vi "process output.vi"(8 "error in":errorcluster, 9 "result allocation":T1, 10 "parameters":T1, 11 "module in":refnum<class "current tag file io module runtime.lvclass">) -> (0 "error out":errorcluster, 1 "results":T1, 2 "parameter allocation":T1, 3 "module out":refnum<class "current tag file io module runtime.lvclass">)   [LabVIEW 2013, in "current tag file io module runtime.lvclass"]
doc: "Provides an interface for information processing by a module at runtime. While this interface performs no operations, a child should provide an override which may process data in any manner necessary."
uses:
  current tag file io module runtime.lvclass
  <vilib>/NI/Tag Bus/table/data table.lvlib
  <vilib>/NI/Tag Bus/table/data polymorphs/read one/read Double.vi
  <vilib>/NI/Tag Bus/table/data polymorphs/write one/write Double.vi
  <vilib>/NI/Tag Bus/table/data polymorphs/read one/read Boolean.vi
  <vilib>/NI/Tag Bus/table/data polymorphs/write one/write Array of String.vi
  <vilib>/NI/Tag Bus/table/data polymorphs/read one/read Array of String.vi
  <vilib>/NI/Tag Bus/table/data polymorphs/read one/read Single.vi
  <vilib>/NI/Tag Bus/table/data polymorphs/write one/write Single.vi
  <vilib>/NI/Tag Bus/table/data polymorphs/read one/read I64.vi
  <vilib>/NI/Tag Bus/table/data polymorphs/write one/write I64.vi
  <vilib>/NI/Tag Bus/table/data polymorphs/read one/read I32.vi
  <vilib>/NI/Tag Bus/table/data polymorphs/write one/write I32.vi
  <vilib>/NI/Tag Bus/table/data polymorphs/read one/read I16.vi
  <vilib>/NI/Tag Bus/table/data polymorphs/write one/write I16.vi
  <vilib>/NI/Tag Bus/table/data polymorphs/read one/read I8.vi
  <vilib>/NI/Tag Bus/table/data polymorphs/write one/write I8.vi
  <vilib>/NI/Tag Bus/table/data polymorphs/read one/read U64.vi
  <vilib>/NI/Tag Bus/table/data polymorphs/write one/write U64.vi
  <vilib>/NI/Tag Bus/table/data polymorphs/read one/read U32.vi
  <vilib>/NI/Tag Bus/table/data polymorphs/write one/write U32.vi
  <vilib>/NI/Tag Bus/table/data polymorphs/read one/read U16.vi
  <vilib>/NI/Tag Bus/table/data polymorphs/write one/write U16.vi
  <vilib>/NI/Tag Bus/table/data polymorphs/read one/read U8.vi
  <vilib>/NI/Tag Bus/table/data polymorphs/write one/write U8.vi
  <vilib>/NI/Tag Bus/table/data polymorphs/write one/write Boolean.vi
  <vilib>/NI/Tag Bus/table/data polymorphs/read one/read String.vi
  <vilib>/NI/Tag Bus/table/data polymorphs/write one/write String.vi
  <vilib>/NI/Tag Bus/table/data polymorphs/read one/read Array of Double.vi
  <vilib>/NI/Tag Bus/table/data polymorphs/write one/write Array of Double.vi
  <vilib>/NI/Tag Bus/table/data polymorphs/read one/read Array of Single.vi
  <vilib>/NI/Tag Bus/table/data polymorphs/write one/write Array of Single.vi
  <vilib>/NI/Tag Bus/table/data polymorphs/read one/read Array of I64.vi
  <vilib>/NI/Tag Bus/table/data polymorphs/write one/write Array of I64.vi
  <vilib>/NI/Tag Bus/table/data polymorphs/read one/read Array of I32.vi
  <vilib>/NI/Tag Bus/table/data polymorphs/write one/write Array of I32.vi
  <vilib>/NI/Tag Bus/table/data polymorphs/read one/read Array of I16.vi
  <vilib>/NI/Tag Bus/table/data polymorphs/write one/write Array of I16.vi
  <vilib>/NI/Tag Bus/table/data polymorphs/read one/read Array of I8.vi
  <vilib>/NI/Tag Bus/table/data polymorphs/write one/write Array of I8.vi
  <vilib>/NI/Tag Bus/table/data polymorphs/read one/read Array of U64.vi
  <vilib>/NI/Tag Bus/table/data polymorphs/write one/write Array of U64.vi
  <vilib>/NI/Tag Bus/table/data polymorphs/read one/read Array of U32.vi
  <vilib>/NI/Tag Bus/table/data polymorphs/write one/write Array of U32.vi
  <vilib>/NI/Tag Bus/table/data polymorphs/read one/read Array of U16.vi
  <vilib>/NI/Tag Bus/table/data polymorphs/write one/write Array of U16.vi
  <vilib>/NI/Tag Bus/table/data polymorphs/read one/read Array of U8.vi
  <vilib>/NI/Tag Bus/table/data polymorphs/write one/write Array of U8.vi
  <vilib>/NI/Tag Bus/table/data polymorphs/read one/read Array of Boolean.vi
  <vilib>/NI/Tag Bus/table/data polymorphs/write one/write Array of Boolean.vi
  <vilib>/NI/Tag Bus/table/data table.ctl
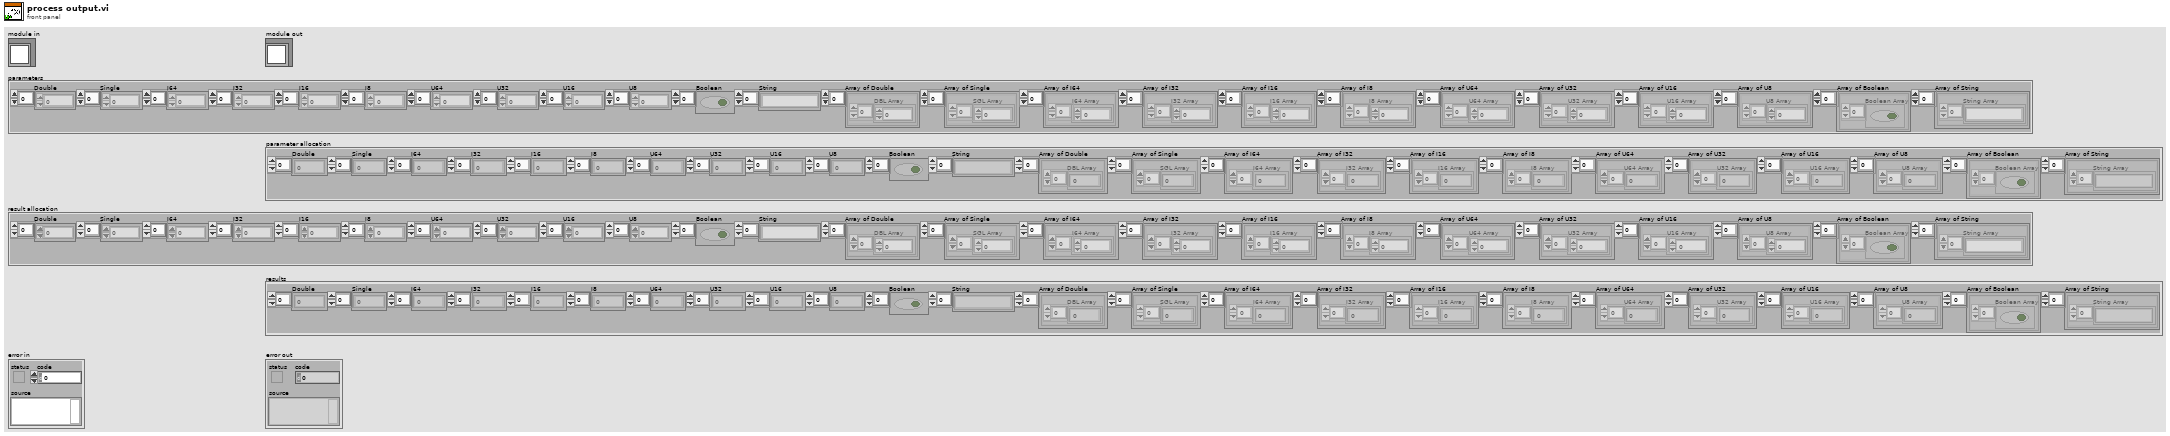
[diagram p1: front panel]
types:
  T1 = typedef "tag bus.lvlib/data table.lvlib/data table.ctl" = cluster{"Double":dbl[], "Single":sgl[], "I64":i64[], "I32":i32[], "I16":i16[], "I8":i8[], "U64":u64[], "U32":u32[], "U16":u16[], "U8":u8[], "Boolean":bool[], "String":string[], "Array of Double":cluster{"DBL Array":dbl[]}[], "Array of Single":cluster{"SGL Array":sgl[]}[], "Array of I64":cluster{"I64 Array":i64[]}[], "Array of I32":cluster{"I32 Array":i32[]}[], "Array of I16":cluster{"I16 Array":i16[]}[], "Array of I8":cluster{"I8 Array":i8[]}[], "Array of U64":cluster{"U64 Array":u64[]}[], "Array of U32":cluster{"U32 Array":u32[]}[], "Array of U16":cluster{"U16 Array":u16[]}[], "Array of U8":cluster{"U8 Array":u8[]}[], "Array of Boolean":cluster{"Boolean Array":bool[]}[], "Array of String":cluster{"String Array":string[]}[]}
  T2 = typedef "current tag file io module runtime.lvclass/runtime tag select configuration.ctl" = cluster{"channel index":i32, "data type":T3}
  T3 = typedef "tag bus.lvlib/tag descriptor.lvclass/Data Type.ctl" = enum16{"Double", "Single", "I64", "I32", "I16", "I8", "U64", "U32", "U16", "U8", "Boolean", "String", "Array of Double", "Array of Single", "Array of I64", "Array of I32", "Array of I16", "Array of I8", "Array of U64", "Array of U32", "Array of U16", "Array of U8", "Array of Boolean", "Array of String"}
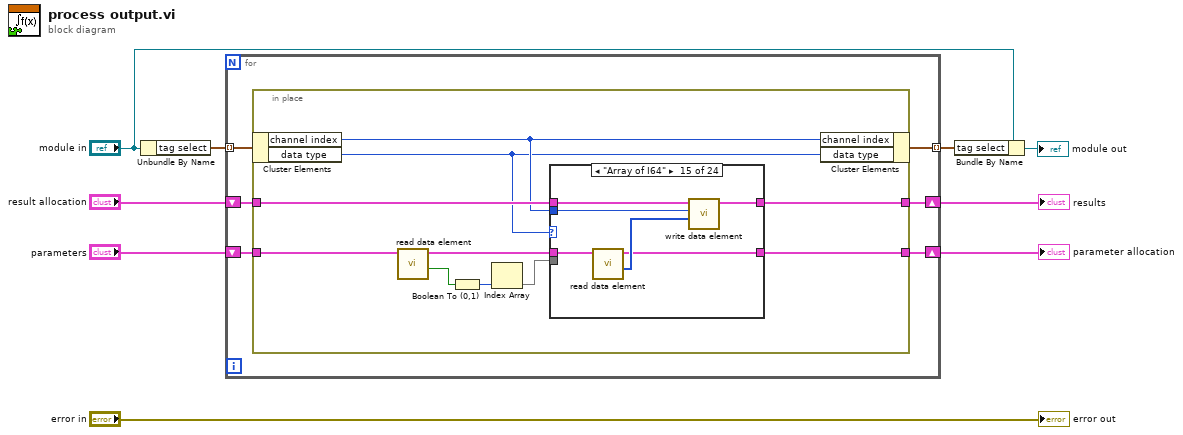
[diagram p0: block diagram]
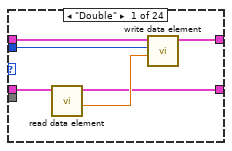
[diagram p2: hidden frame]
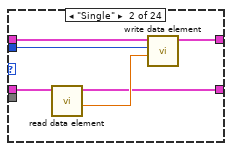
[diagram p3: hidden frame]
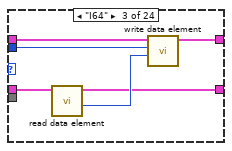
[diagram p4: hidden frame]
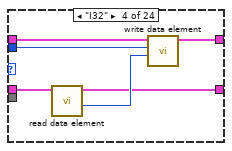
[diagram p5: hidden frame]
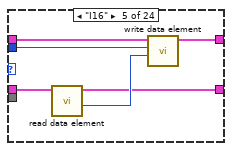
[diagram p6: hidden frame]
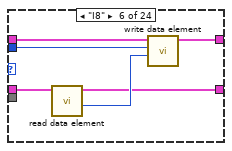
[diagram p7: hidden frame]
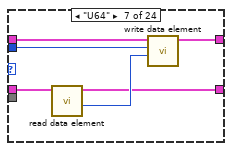
[diagram p8: hidden frame]
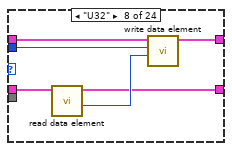
[diagram p9: hidden frame]
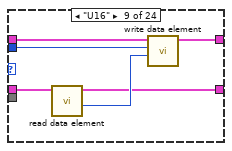
[diagram p10: hidden frame]
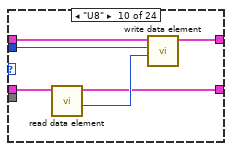
[diagram p11: hidden frame]
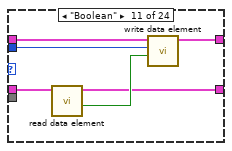
[diagram p12: hidden frame]
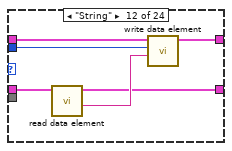
[diagram p13: hidden frame]
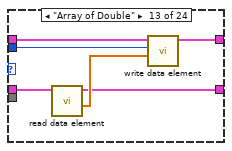
[diagram p14: hidden frame]
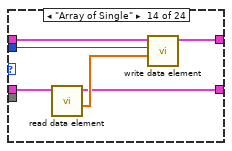
[diagram p15: hidden frame]
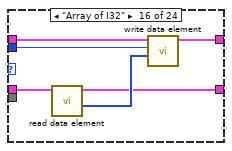
[diagram p16: hidden frame]
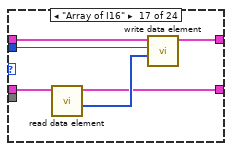
[diagram p17: hidden frame]
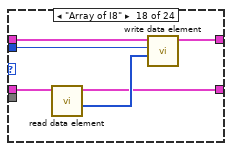
[diagram p18: hidden frame]
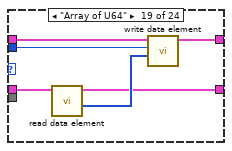
[diagram p19: hidden frame]
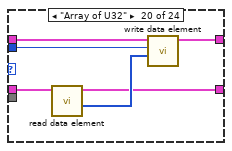
[diagram p20: hidden frame]
diagram:
  n1 = Unbundle By Name("module in") -> ("tag select"=w7:T2[])
  n2 = for {
    tunnel: w7 -> [w15] mode=indexing
    tunnel: [w14] -> w6 mode=indexing
    shift-right: [w10] -> w4
    shift-left: "parameters" -> [w13]
    shift-right: [w11] -> w2
    shift-left: "result allocation" -> [w12]
    n3 = in-place {
      in-place-border: w13 -> [w25]
      in-place-border: w12 -> [w24]
      in-place-border: [w23] -> w11
      in-place-border: [w18] -> w10
      n4 = in-place-cluster #1(w15) -> ("channel index"=w17:i32, "data type"=w16:T3)
      n5 = call-poly <vilib>:"read data element.vi"("data table in"=w25) -> ("value"=w21:bool, "data table out"=w19:T1)  [unwired: 9 in]
      n6 = Boolean To (0,1)(Boolean=w21) -> (0, 1=w22:i16)
      n7 = Index Array(index=w22) -> (element=w20)  [unwired: 1 in]
      n8 = case shown="\"Array of I64\"" w16 {
        tunnel: w24 -> [w26 w32 w38 w44 w50 w56 w62 w68 w74 w80 w86 w92 w98 w104 w110 w116 w122 w128 w134 w140 w146 w152 w158 w164]
        tunnel: [w31 w37 w43 w49 w55 w61 w67 w73 w79 w85 w91 w97 w103 w109 w115 w121 w127 w133 w139 w145 w151 w157 w163 w169] -> w23
        tunnel: w20 -> [_ _ _ _ _ _ _ _ _ _ _ _ _ _ _ _ _ _ _ _ _ _ _ _]
        tunnel: w17 -> [w30 w36 w42 w48 w54 w60 w66 w72 w78 w84 w90 w96 w102 w108 w114 w120 w126 w132 w138 w144 w150 w156 w162 w168]
        tunnel: w19 -> [w28 w34 w40 w46 w52 w58 w64 w70 w76 w82 w88 w94 w100 w106 w112 w118 w124 w130 w136 w142 w148 w154 w160 w166]
        tunnel: [w27 w33 w39 w45 w51 w57 w63 w69 w75 w81 w87 w93 w99 w105 w111 w117 w123 w129 w135 w141 w147 w153 w159 w165] -> w18
        frame "Double" {
          n9 = call-poly <vilib>:"read data element.vi"("data table in"=w28) -> ("value"=w29:dbl, "data table out"=w27:T1)  [unwired: 9 in]
          n10 = call-poly <vilib>:"write data element.vi"("value"=w29, "index"=w30, "data table in"=w26) -> ("data table out"=w31:T1)  [unwired: 8 in]
        }
        frame "Single" {
          n11 = call-poly <vilib>:"read data element.vi"("data table in"=w34) -> ("value"=w35:sgl, "data table out"=w33:T1)  [unwired: 9 in]
          n12 = call-poly <vilib>:"write data element.vi"("value"=w35, "index"=w36, "data table in"=w32) -> ("data table out"=w37:T1)  [unwired: 8 in]
        }
        frame "I64" {
          n13 = call-poly <vilib>:"read data element.vi"("data table in"=w40) -> ("value"=w41:i64, "data table out"=w39:T1)  [unwired: 9 in]
          n14 = call-poly <vilib>:"write data element.vi"("value"=w41, "index"=w42, "data table in"=w38) -> ("data table out"=w43:T1)  [unwired: 8 in]
        }
        frame "I32" {
          n15 = call-poly <vilib>:"read data element.vi"("data table in"=w46) -> ("value"=w47:i32, "data table out"=w45:T1)  [unwired: 9 in]
          n16 = call-poly <vilib>:"write data element.vi"("value"=w47, "index"=w48, "data table in"=w44) -> ("data table out"=w49:T1)  [unwired: 8 in]
        }
        frame "I16" {
          n17 = call-poly <vilib>:"read data element.vi"("data table in"=w52) -> ("value"=w53:i16, "data table out"=w51:T1)  [unwired: 9 in]
          n18 = call-poly <vilib>:"write data element.vi"("value"=w53, "index"=w54, "data table in"=w50) -> ("data table out"=w55:T1)  [unwired: 8 in]
        }
        frame "I8" {
          n19 = call-poly <vilib>:"read data element.vi"("data table in"=w58) -> ("value"=w59:i8, "data table out"=w57:T1)  [unwired: 9 in]
          n20 = call-poly <vilib>:"write data element.vi"("value"=w59, "index"=w60, "data table in"=w56) -> ("data table out"=w61:T1)  [unwired: 8 in]
        }
        frame "U64" {
          n21 = call-poly <vilib>:"read data element.vi"("data table in"=w64) -> ("value"=w65:u64, "data table out"=w63:T1)  [unwired: 9 in]
          n22 = call-poly <vilib>:"write data element.vi"("value"=w65, "index"=w66, "data table in"=w62) -> ("data table out"=w67:T1)  [unwired: 8 in]
        }
        frame "U32" {
          n23 = call-poly <vilib>:"read data element.vi"("data table in"=w70) -> ("value"=w71:u32, "data table out"=w69:T1)  [unwired: 9 in]
          n24 = call-poly <vilib>:"write data element.vi"("value"=w71, "index"=w72, "data table in"=w68) -> ("data table out"=w73:T1)  [unwired: 8 in]
        }
        frame "U16" {
          n25 = call-poly <vilib>:"read data element.vi"("data table in"=w76) -> ("value"=w77:u16, "data table out"=w75:T1)  [unwired: 9 in]
          n26 = call-poly <vilib>:"write data element.vi"("value"=w77, "index"=w78, "data table in"=w74) -> ("data table out"=w79:T1)  [unwired: 8 in]
        }
        frame "U8" {
          n27 = call-poly <vilib>:"read data element.vi"("data table in"=w82) -> ("value"=w83:u8, "data table out"=w81:T1)  [unwired: 9 in]
          n28 = call-poly <vilib>:"write data element.vi"("value"=w83, "index"=w84, "data table in"=w80) -> ("data table out"=w85:T1)  [unwired: 8 in]
        }
        frame "Boolean" {
          n29 = call-poly <vilib>:"read data element.vi"("data table in"=w88) -> ("value"=w89:bool, "data table out"=w87:T1)  [unwired: 9 in]
          n30 = call-poly <vilib>:"write data element.vi"("value"=w89, "index"=w90, "data table in"=w86) -> ("data table out"=w91:T1)  [unwired: 8 in]
        }
        frame "String" {
          n31 = call-poly <vilib>:"read data element.vi"("data table in"=w94) -> ("value"=w95:string, "data table out"=w93:T1)  [unwired: 9 in]
          n32 = call-poly <vilib>:"write data element.vi"("value"=w95, "index"=w96, "data table in"=w92) -> ("data table out"=w97:T1)  [unwired: 8 in]
        }
        frame "Array of Double" {
          n33 = call-poly <vilib>:"read data element.vi"("data table in"=w100) -> ("value"=w101:dbl[], "data table out"=w99:T1)  [unwired: 9 in]
          n34 = call-poly <vilib>:"write data element.vi"("value"=w101, "index"=w102, "data table in"=w98) -> ("data table out"=w103:T1)  [unwired: 8 in]
        }
        frame "Array of Single" {
          n35 = call-poly <vilib>:"read data element.vi"("data table in"=w106) -> ("value"=w107:sgl[], "data table out"=w105:T1)  [unwired: 9 in]
          n36 = call-poly <vilib>:"write data element.vi"("value"=w107, "index"=w108, "data table in"=w104) -> ("data table out"=w109:T1)  [unwired: 8 in]
        }
        frame "Array of I64" {
          n37 = call-poly <vilib>:"read data element.vi"("data table in"=w112) -> ("value"=w113:i64[], "data table out"=w111:T1)  [unwired: 9 in]
          n38 = call-poly <vilib>:"write data element.vi"("value"=w113, "index"=w114, "data table in"=w110) -> ("data table out"=w115:T1)  [unwired: 8 in]
        }
        frame "Array of I32" {
          n39 = call-poly <vilib>:"read data element.vi"("data table in"=w118) -> ("value"=w119:i32[], "data table out"=w117:T1)  [unwired: 9 in]
          n40 = call-poly <vilib>:"write data element.vi"("value"=w119, "index"=w120, "data table in"=w116) -> ("data table out"=w121:T1)  [unwired: 8 in]
        }
        frame "Array of I16" {
          n41 = call-poly <vilib>:"read data element.vi"("data table in"=w124) -> ("value"=w125:i16[], "data table out"=w123:T1)  [unwired: 9 in]
          n42 = call-poly <vilib>:"write data element.vi"("value"=w125, "index"=w126, "data table in"=w122) -> ("data table out"=w127:T1)  [unwired: 8 in]
        }
        frame "Array of I8" {
          n43 = call-poly <vilib>:"read data element.vi"("data table in"=w130) -> ("value"=w131:i8[], "data table out"=w129:T1)  [unwired: 9 in]
          n44 = call-poly <vilib>:"write data element.vi"("value"=w131, "index"=w132, "data table in"=w128) -> ("data table out"=w133:T1)  [unwired: 8 in]
        }
        frame "Array of U64" {
          n45 = call-poly <vilib>:"read data element.vi"("data table in"=w136) -> ("value"=w137:u64[], "data table out"=w135:T1)  [unwired: 9 in]
          n46 = call-poly <vilib>:"write data element.vi"("value"=w137, "index"=w138, "data table in"=w134) -> ("data table out"=w139:T1)  [unwired: 8 in]
        }
        frame "Array of U32" {
          n47 = call-poly <vilib>:"read data element.vi"("data table in"=w142) -> ("value"=w143:u32[], "data table out"=w141:T1)  [unwired: 9 in]
          n48 = call-poly <vilib>:"write data element.vi"("value"=w143, "index"=w144, "data table in"=w140) -> ("data table out"=w145:T1)  [unwired: 8 in]
        }
        frame "Array of U16" {
          n49 = call-poly <vilib>:"read data element.vi"("data table in"=w148) -> ("value"=w149:u16[], "data table out"=w147:T1)  [unwired: 9 in]
          n50 = call-poly <vilib>:"write data element.vi"("value"=w149, "index"=w150, "data table in"=w146) -> ("data table out"=w151:T1)  [unwired: 8 in]
        }
        frame "Array of U8" {
          n51 = call-poly <vilib>:"read data element.vi"("data table in"=w154) -> ("value"=w155:u8[], "data table out"=w153:T1)  [unwired: 9 in]
          n52 = call-poly <vilib>:"write data element.vi"("value"=w155, "index"=w156, "data table in"=w152) -> ("data table out"=w157:T1)  [unwired: 8 in]
        }
        frame "Array of Boolean" {
          n53 = call-poly <vilib>:"read data element.vi"("data table in"=w160) -> ("value"=w161:bool[], "data table out"=w159:T1)  [unwired: 9 in]
          n54 = call-poly <vilib>:"write data element.vi"("value"=w161, "index"=w162, "data table in"=w158) -> ("data table out"=w163:T1)  [unwired: 8 in]
        }
        frame "Array of String" {
          n55 = call-poly <vilib>:"read data element.vi"("data table in"=w166) -> ("value"=w167:string[], "data table out"=w165:T1)  [unwired: 9 in]
          n56 = call-poly <vilib>:"write data element.vi"("value"=w167, "index"=w168, "data table in"=w164) -> ("data table out"=w169:T1)  [unwired: 8 in]
        }
      }
      n57 = in-place-cluster #1("channel index"=w17, "data type"=w16) -> (w14:T2)
    }
  }
  "results" <- w2
  "parameter allocation" <- w4
  n58 = Bundle By Name(cluster="module in", "tag select"=w6) -> (→"module out":refnum<class "current tag file io module runtime.lvclass">)
  "error out" <- "error in"
